vi "Resize and Position Bundle By Name.vi"(7 "Sources":refnum<vi>[](array[refnum]), 8 "error in":errorcluster, 9 "BBN Node":refnum<vi>, 10 "Vertical Center":i32, 11 "Right":i16) -> (0 "error out":errorcluster)   [LabVIEW 2012, in "Build Cluster of References__RCF.lvlib"]
uses:
  Build Cluster of References__RCF.lvlib
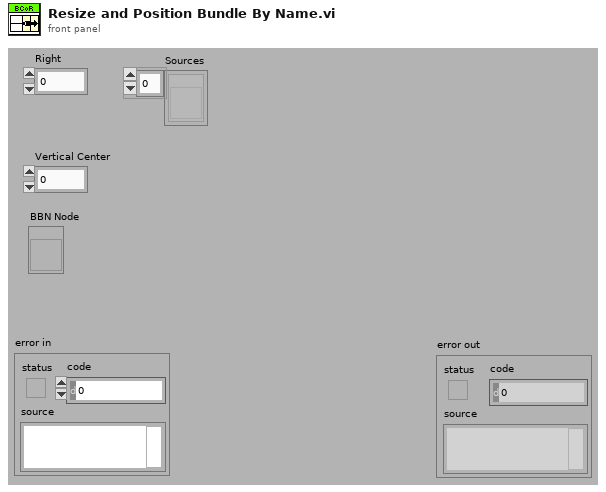
[diagram p1: front panel]
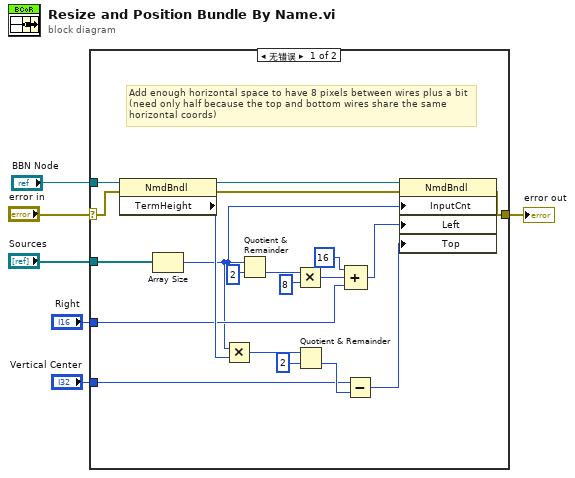
[diagram p0: block diagram]
diagram:
  n1 = case shown="无错误" "error in" {
    selector: "error in" -> [w11 w27]
    tunnel: "Sources" -> [w20 _]
    tunnel: "BBN Node" -> [w17 _]
    tunnel: [w8 w27] -> w1
    tunnel: "Vertical Center" -> [w16 _]
    tunnel: "Right" -> [w12 _]
    frame No Error {
      # "Add enough horizontal space to have 8 pixels between wires plus a bit (need only half because the top and bottom wires share the same horizontal coords)"
      n2 = property class="NmdBndl"(reference=w17, error in=w11) -> (reference out=w15:refnum<vi>, error out=w14:errorcluster, "TermHeight"=w24:i32)
      n3 = Array Size(array=w20) -> (size(s)=w7:i32)
      n4 = Multiply(x=w7, y=w24) -> (x*y=w22:i32)
      n5 = Quotient & Remainder(x=w7, y=2) -> (floor(x/y)=w13:i32)  [unwired: 1 out]
      n6 = Multiply(x=w13, y=8 ("x")) -> (x*y=w19:i32)
      n7 = Quotient & Remainder(x=w22, y=2) -> (floor(x/y)=w21:i32)  [unwired: 1 out]
      n8 = Compound Arithmetic op=ADD(16 ("value"), w19, w12) -> (w10:i32)
      n9 = Subtract(x=w16, y=w21) -> (x-y=w9:i32)
      n10 = property class="NmdBndl"(reference=w15, error in=w14, "InputCnt"=w7, "Left"=w10, "Top"=w9) -> (error out=w8:errorcluster)  [unwired: 1 out]
    }
    frame Error {
    }
  }
  "error out" <- w1
